vi "Config - merge.vi"(8 "error in (no error)":errorcluster) -> (0 "error out":errorcluster)   [LabVIEW 2026]
doc: "Unit test (Caraya) for launch-config resolution.\nWith no config path the effective config equals the baseline inputs; a defined-but-missing path returns a non-fatal warning and falls back to the baseline; a present-but-invalid file (unparseable or schema-invalid) fails launch with no fallback.\nThe no-path and missing-path cases need no file; the invalid-file cases use a temp-root fixture that writes a malformed and a schema-invalid JSON file. Each expected error is captured and cleared per case.\n\nImplements LMBR-T-020, T-022, T-023 -> SRS-044, SRS-047, SRS-048. Assert-level IDs: Test-ID-Assert-Checklist.md."
uses:
  <vilib>/addons/_JKI Toolkits/Caraya/classes/Test/Test.lvclass
  src/Lumberjack.lvlib
  src/TypeDefs/ConfigDTO/FilterDTO.ctl
  src/TypeDefs/ConfigDTO/AppenderConfigDTO.ctl
  src/TypeDefs/ConfigDTO/FileConfigDTO.ctl
  src/TypeDefs/ConfigDTO/FileAppenderConfigDTO.ctl
  src/TypeDefs/ConfigDTO/LumberjackConfigDTO.ctl
  <vilib>/addons/_JKI Toolkits/Caraya/classes/Assert/Assert.lvclass
  <vilib>/addons/_JKI Toolkits/Caraya/classes/Assert/Assert Equal Value_Variant.vi
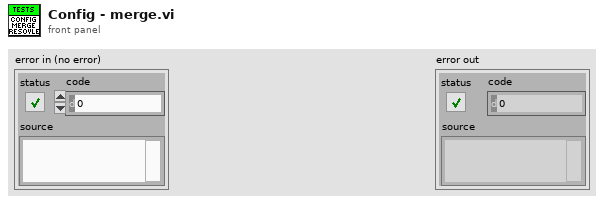
[diagram p1: front panel]
types:
  T1 = typedef "Lumberjack.lvlib/LumberjackConfigDTO.ctl" = cluster{"schemaVersion":string, "globalThreshold":string, "defaultFileAppender":T2}
  T2 = typedef "Lumberjack.lvlib/FileAppenderConfigDTO.ctl" = cluster{"common":T3, "file":T5}
  T3 = typedef "Lumberjack.lvlib/AppenderConfigDTO.ctl" = cluster{"id":string, "threshold":string, "filter":T4, "queueBound":i32, "dropPolicy":string, "useUTC":bool}
  T4 = typedef "Lumberjack.lvlib/FilterDTO.ctl" = cluster{"mode":string, "levelMin":string, "levelMax":string, "tagPrefix":string}
  T5 = typedef "Lumberjack.lvlib/FileConfigDTO.ctl" = cluster{"rootFolder":string, "maxFileSize":i64, "maxFileCount":i32, "baseName":string, "extension":string, "delimiter":string, "calendarFolderTree":bool}
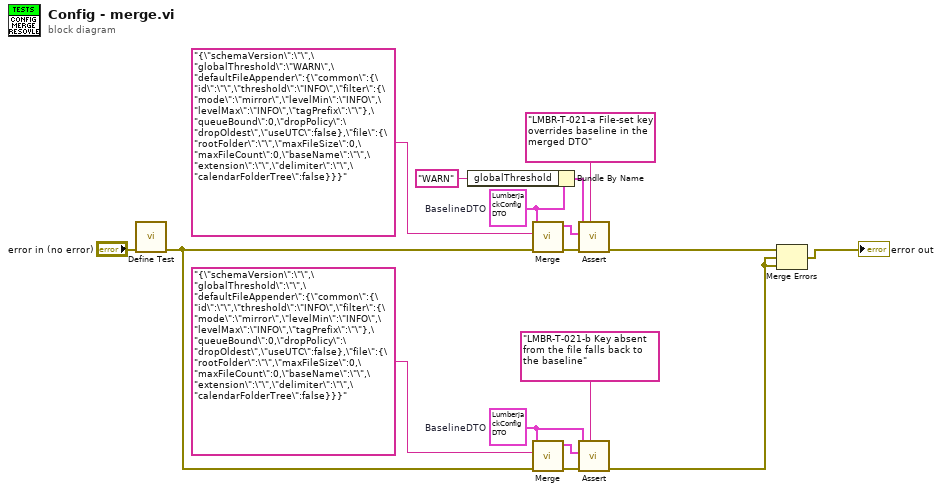
[diagram p0: block diagram]
diagram:
  w2 = T1 {"schemaVersion"="", "globalThreshold"="INFO", "defaultFileAppender"={"common"={"id"="", "threshold"="INFO", "filter"={"mode"="mirror", "levelMin"="INFO", "levelMax"="INFO", "tagPrefix"=""}, "queueBound"=0, "dropPolicy"="dropOldest", "useUTC"=FALSE}, "file"={"rootFolder"="", "maxFileSize"=0, "maxFileCount"=0, "baseName"="", "extension"="", "delimiter"="", "calendarFolderTree"=FALSE}}}  # BaselineDTO
  w14 = T1 {"schemaVersion"="", "globalThreshold"="INFO", "defaultFileAppender"={"common"={"id"="", "threshold"="INFO", "filter"={"mode"="mirror", "levelMin"="INFO", "levelMax"="INFO", "tagPrefix"=""}, "queueBound"=0, "dropPolicy"="dropOldest", "useUTC"=FALSE}, "file"={"rootFolder"="", "maxFileSize"=0, "maxFileCount"=0, "baseName"="", "extension"="", "delimiter"="", "calendarFolderTree"=FALSE}}}  # BaselineDTO
  n1 = call <vilib>:"Define Test.vi"("error in (no error)"="error in (no error)") -> ("error out"=w3:errorcluster)  [unwired: 9 in, 1 out]
  n2 = Bundle By Name(cluster=w14, "globalThreshold"="WARN") -> (w12:T1)
  n3 = call "Merge.vi"("error in (no error)"=w3, "JSONText"="{\"schemaVersion\":\"\",\"globalThreshold\":\"WARN\",\"defaultFileAppender\":{\"common\":{\"id\":\"\",\"threshold\":\"INFO\",\"filter\":{\"mode\":\"mirror\",\"levelMin\":\"INFO\",\"levelMax\":\"INFO\",\"tagPrefix\":\"\"},\"queueBound\":0,\"dropPolicy\":\"dropOldest\",\"useUTC\":false},\"file\":{\"rootFolder\":\"\",\"maxFileSize\":0,\"maxFileCount\":0,\"baseName\":\"\",\"extension\":\"\",\"delimiter\":\"\",\"calendarFolderTree\":false}}}", "BaselineDTO"=w14) -> ("error out"=w15:errorcluster, "MergedDTO"=w11:T1)  [unwired: 7 in]
  n4 = call "Merge.vi"("error in (no error)"=w3, "JSONText"="{\"schemaVersion\":\"\",\"globalThreshold\":\"\",\"defaultFileAppender\":{\"common\":{\"id\":\"\",\"threshold\":\"INFO\",\"filter\":{\"mode\":\"mirror\",\"levelMin\":\"INFO\",\"levelMax\":\"INFO\",\"tagPrefix\":\"\"},\"queueBound\":0,\"dropPolicy\":\"dropOldest\",\"useUTC\":false},\"file\":{\"rootFolder\":\"\",\"maxFileSize\":0,\"maxFileCount\":0,\"baseName\":\"\",\"extension\":\"\",\"delimiter\":\"\",\"calendarFolderTree\":false}}}", "BaselineDTO"=w2) -> ("error out"=w6:errorcluster, "MergedDTO"=w5:T1)  [unwired: 7 in]
  n5 = call-poly <vilib>:"Assert.vi"("Label"="LMBR-T-021-a File-set key overrides baseline in the merged DTO", "error in (no error)"=w15, "Actual"=w11, "Expected"=w12) -> ("error out"=w10:errorcluster)  [unwired: 6 in, 1 out]
  n6 = call-poly <vilib>:"Assert.vi"("Label"="LMBR-T-021-b Key absent from the file falls back to the baseline", "error in (no error)"=w6, "Actual"=w5, "Expected"=w2) -> ("error out"=w1:errorcluster)  [unwired: 6 in, 1 out]
  n7 = Merge Errors(w10, w1, w1) -> (→"error out":errorcluster)
